vi "Numero y su inverso.vi"() -> ()   [LabVIEW 2019]
panel:
  out "Numeric 2":dbl
  out "Numeric":dbl
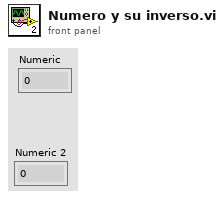
[diagram p1: front panel]
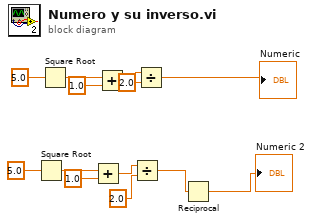
[diagram p0: block diagram]
diagram:
  n1 = Square Root(x=5.0) -> (sqrt(x)=w4:dbl)
  n2 = Square Root(x=5.0) -> (sqrt(x)=w12:dbl)
  n3 = Add(x=w4, y=1.0) -> (x+y=w6:dbl)
  n4 = Add(x=w12, y=1.0) -> (x+y=w10:dbl)
  n5 = Divide(x=w6, y=2.0) -> (x/y=w2:dbl)
  n6 = Divide(x=w10, y=2.0) -> (x/y=→"Numeric":dbl)
  n7 = Reciprocal(x=w2) -> (1/x=→"Numeric 2":dbl)
